vi "XLP80_Action_ErrorCodeMessage_FCCU_Errors.vi"(9 "TimeStamp":dbl format="%.2f", 11 "SYS_Error_Name":string) -> (3 "message string":string)   [LabVIEW 2021]
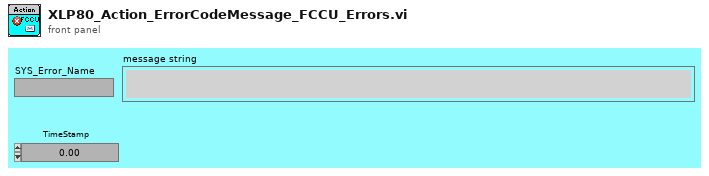
[diagram p1: front panel]
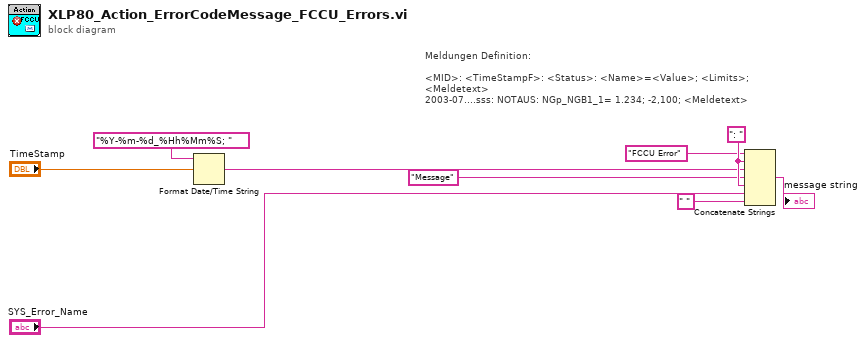
[diagram p0: block diagram]
diagram:
  w9 = ": " ("string")
  # "Meldungen Definition:\n\n<MID>: <TimeStampF>: <Status>: <Name>=<Value>; <Limits>; <Meldetext>\n2003-07....sss: NOTAUS: NGp_NGB1_1= 1.234; -2,100; <Meldetext>"
  n1 = Format Date/Time String(time format string (%c)="%Y-%m-%d_%Hh%Mm%S; ", seconds (now)="TimeStamp") -> (date/time string=w5:string)  [unwired: 1 in]
  n2 = Concatenate Strings("FCCU Error" ("string"), w9, w5, "Message" ("Ring Text.Text"), w9, "SYS_Error_Name", " " ("string")) -> (→"message string":string)
